vi "获取硬盘ID和主板ID.vi"() -> ()   [LabVIEW 2015]
panel:
  out "standard output 2":string caption="硬盘ID"
  out "standard output":string caption="主板ID"
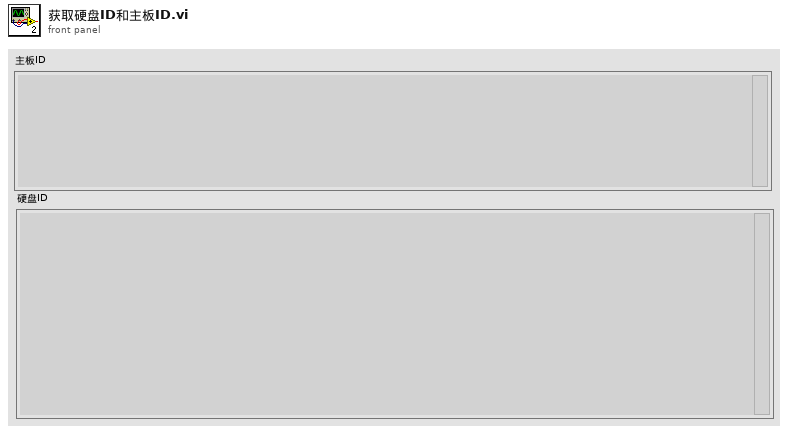
[diagram p1: front panel]
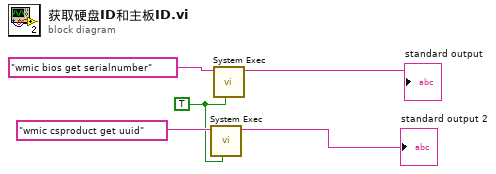
[diagram p0: block diagram]
diagram:
  w2 = TRUE ("run minimized? (F)")
  n1 = call <vilib>:"System Exec.vi"("run minimized? (F)"=w2, "command line"="wmic csproduct get uuid") -> ("standard output"=→"standard output 2":string)  [unwired: 6 in, 3 out]
  n2 = call <vilib>:"System Exec.vi"("run minimized? (F)"=w2, "command line"="wmic bios get serialnumber") -> ("standard output"=→"standard output":string)  [unwired: 6 in, 3 out]
